vi "Start Rx.vi"(6 "error in (no error)":errorcluster, 8 "RX PARAMETER PANEL":T1={"Chain Mask"=0, "CF(MHz)"=2412, "CF2(MHz)"=0, "Data Rate"=0} {"Chain Mask" items=["0x1 : ch0"=1, "0x2 : ch1"=2, "0x4 : ch2"=4, "0x8 : ch3"=8, "0x3 : ch0, ch1"=3, "0x7 : ch0, ch1, ch2"=7, "0x15 : ch0, ch1, ch2, ch3"=15, "0x5 : ch0, ch2"=5, "0x10 : ch1, ch3"=10, "0x9 : ch1, ch3"=9, "0x12 : ch2, ch4"=12]; "Data Rate" items=["RATE_11B_LONG_1_MBPS"=0, "RATE_11B_LONG_2_MBPS"=1, "RATE_11B_LONG_5_5_MBPS"=2, "RATE_11B_LONG_11_MBPS"=3, "RATE_11B_SHORT_2_MBPS"=4, "RATE_11B_SHORT_5_5_MBPS"=5, "RATE_11B_SHORT_11_MBPS"=6, "RATE_11A_6_MBPS"=7, "RATE_11A_9_MBPS"=8, "RATE_11A_12_MBPS"=9, "RATE_11A_18_MBPS"=10, "RATE_11A_24_MBPS"=11, "RATE_11A_36_MBPS"=12, "RATE_11A_48_MBPS"=13, "RATE_11A_54_MBPS"=14, "RATE_11N_HT20_MCS0"=15, "RATE_11N_HT20_MCS1"=16, "RATE_11N_HT20_MCS2"=17, "RATE_11N_HT20_MCS3"=18, "RATE_11N_HT20_MCS4"=19, "RATE_11N_HT20_MCS5"=20, "RATE_11N_HT20_MCS6"=21, "RATE_11N_HT20_MCS7"=22, "RATE_11N_HT40_MCS0"=23, "RATE_11N_HT40_MCS1"=24, "RATE_11N_HT40_MCS2"=25, "RATE_11N_HT40_MCS3"=26, "RATE_11N_HT40_MCS4"=27, "RATE_11N_HT40_MCS5"=28, "RATE_11N_HT40_MCS6"=29, "RATE_11N_HT40_MCS7"=30, "RATE_11AC_HT20_MCS0"=31, "RATE_11AC_HT20_MCS1"=32, "RATE_11AC_HT20_MCS2"=33, "RATE_11AC_HT20_MCS3"=34, "RATE_11AC_HT20_MCS4"=35, "RATE_11AC_HT20_MCS5"=36, "RATE_11AC_HT20_MCS6"=37, "RATE_11AC_HT20_MCS7"=38, "RATE_11AC_HT20_MCS8"=39, "RATE_11AC_HT20_MCS9"=40, "RATE_11AC_HT40_MCS0"=41, "RATE_11AC_HT40_MCS1"=42, "RATE_11AC_HT40_MCS2"=43, "RATE_11AC_HT40_MCS3"=44, "RATE_11AC_HT40_MCS4"=45, "RATE_11AC_HT40_MCS5"=46, "RATE_11AC_HT40_MCS6"=47, "RATE_11AC_HT40_MCS7"=48, "RATE_11AC_HT40_MCS8"=49, "RATE_11AC_HT40_MCS9"=50, "RATE_11AC_HT80_MCS0"=51, "RATE_11AC_HT80_MCS1"=52, "RATE_11AC_HT80_MCS2"=53, "RATE_11AC_HT80_MCS3"=54, "RATE_11AC_HT80_MCS4"=55, "RATE_11AC_HT80_MCS5"=56, "RATE_11AC_HT80_MCS6"=57, "RATE_11AC_HT80_MCS7"=58, "RATE_11AC_HT80_MCS8"=59, "RATE_11AC_HT80_MCS9"=60, "RATE_11N_HT20_MCS8"=61, "RATE_11N_HT20_MCS9"=62, "RATE_11N_HT20_MCS10"=63, "RATE_11N_HT20_MCS11"=64, "RATE_11N_HT20_MCS12"=65, "RATE_11N_HT20_MCS13"=66, "RATE_11N_HT20_MCS14"=67, "RATE_11N_HT20_MCS15"=68, "RATE_11N_HT40_MCS8"=69, "RATE_11N_HT40_MCS9"=70, "RATE_11N_HT40_MCS10"=71, "RATE_11N_HT40_MCS11"=72, "RATE_11N_HT40_MCS12"=73, "RATE_11N_HT40_MCS13"=74, "RATE_11N_HT40_MCS14"=75, "RATE_11N_HT40_MCS15"=76, "RATE_11AC_HT20_MCS10"=77, "RATE_11AC_HT20_MCS11"=78, "RATE_11AC_HT20_MCS12"=79, "RATE_11AC_HT20_MCS13"=80, "RATE_11AC_HT20_MCS14"=81, "RATE_11AC_HT20_MCS15"=82, "RATE_11AC_HT20_MCS16"=83, "RATE_11AC_HT20_MCS17"=84, "RATE_11AC_HT20_MCS18"=85, "RATE_11AC_HT20_MCS19"=86, "RATE_11AC_HT40_MCS10"=87, "RATE_11AC_HT40_MCS11"=88, "RATE_11AC_HT40_MCS12"=89, "RATE_11AC_HT40_MCS13"=90, "RATE_11AC_HT40_MCS14"=91, "RATE_11AC_HT40_MCS15"=92, "RATE_11AC_HT40_MCS16"=93, "RATE_11AC_HT40_MCS17"=94, "RATE_11AC_HT40_MCS18"=95, "RATE_11AC_HT40_MCS19"=96, "RATE_11AC_HT80_MCS10"=97, "RATE_11AC_HT80_MCS11"=98, "RATE_11AC_HT80_MCS12"=99, "RATE_11AC_HT80_MCS13"=100, "RATE_11AC_HT80_MCS14"=101, "RATE_11AC_HT80_MCS15"=102, "RATE_11AC_HT80_MCS16"=103, "RATE_11AC_HT80_MCS17"=104, "RATE_11AC_HT80_MCS18"=105, "RATE_11AC_HT80_MCS19"=106, "RATE_11N_HT20_MCS16"=107, "RATE_11N_HT20_MCS17"=108, "RATE_11N_HT20_MCS18"=109, "RATE_11N_HT20_MCS19"=110, "RATE_11N_HT20_MCS20"=111, "RATE_11N_HT20_MCS21"=112, "RATE_11N_HT20_MCS22"=113, "RATE_11N_HT20_MCS23"=114, "RATE_11N_HT40_MCS16"=115, "RATE_11N_HT40_MCS17"=116, "RATE_11N_HT40_MCS18"=117, "RATE_11N_HT40_MCS19"=118, "RATE_11N_HT40_MCS20"=119, "RATE_11N_HT40_MCS21"=120, "RATE_11N_HT40_MCS22"=121, "RATE_11N_HT40_MCS23"=122, "RATE_11AC_HT20_MCS20"=123, "RATE_11AC_HT20_MCS21"=124, "RATE_11AC_HT20_MCS22"=125, "RATE_11AC_HT20_MCS23"=126, "RATE_11AC_HT20_MCS24"=127, "RATE_11AC_HT20_MCS25"=128, "RATE_11AC_HT20_MCS26"=129, "RATE_11AC_HT20_MCS27"=130, "RATE_11AC_HT20_MCS28"=131, "RATE_11AC_HT20_MCS29"=132, "RATE_11AC_HT40_MCS20"=133, "RATE_11AC_HT40_MCS21"=134, "RATE_11AC_HT40_MCS22"=135, "RATE_11AC_HT40_MCS23"=136, "RATE_11AC_HT40_MCS24"=137, "RATE_11AC_HT40_MCS25"=138, "RATE_11AC_HT40_MCS26"=139, "RATE_11AC_HT40_MCS27"=140, "RATE_11AC_HT40_MCS28"=141, "RATE_11AC_HT40_MCS29"=142, "RATE_11AC_HT80_MCS20"=143, "RATE_11AC_HT80_MCS21"=144, "RATE_11AC_HT80_MCS22"=145, "RATE_11AC_HT80_MCS23"=146, "RATE_11AC_HT80_MCS24"=147, "RATE_11AC_HT80_MCS25"=148, "RATE_11AC_HT80_MCS26"=149, "RATE_11AC_HT80_MCS27"=150, "RATE_11AC_HT80_MCS28"=151, "RATE_11AC_HT80_MCS29"=152, "RATE_11AC_HT20_MCS30"=153, "RATE_11AC_HT20_MCS31"=154, "RATE_11AC_HT20_MCS32"=155, "RATE_11AC_HT20_MCS33"=156, "RATE_11AC_HT20_MCS34"=157, "RATE_11AC_HT20_MCS35"=158, "RATE_11AC_HT20_MCS36"=159, "RATE_11AC_HT20_MCS37"=160, "RATE_11AC_HT20_MCS38"=161, "RATE_11AC_HT20_MCS39"=162, "RATE_11AC_HT40_MCS30"=163, "RATE_11AC_HT40_MCS31"=164, "RATE_11AC_HT40_MCS32"=165, "RATE_11AC_HT40_MCS33"=166, "RATE_11AC_HT40_MCS34"=167, "RATE_11AC_HT40_MCS35"=168, "RATE_11AC_HT40_MCS36"=169, "RATE_11AC_HT40_MCS37"=170, "RATE_11AC_HT40_MCS38"=171, "RATE_11AC_HT40_MCS39"=172, "RATE_11AC_HT80_MCS30"=173, "RATE_11AC_HT80_MCS31"=174, "RATE_11AC_HT80_MCS32"=175, "RATE_11AC_HT80_MCS33"=176, "RATE_11AC_HT80_MCS34"=177, "RATE_11AC_HT80_MCS35"=178, "RATE_11AC_HT80_MCS36"=179, "RATE_11AC_HT80_MCS37"=180, "RATE_11AC_HT80_MCS38"=181, "RATE_11AC_HT80_MCS39"=182, "RATE_11AC_HT160_MCS0"=183, "RATE_11AC_HT160_MCS1"=184, "RATE_11AC_HT160_MCS2"=185, "RATE_11AC_HT160_MCS3"=186, "RATE_11AC_HT160_MCS4"=187, "RATE_11AC_HT160_MCS5"=188, "RATE_11AC_HT160_MCS6"=189, "RATE_11AC_HT160_MCS7"=190, "RATE_11AC_HT160_MCS8"=191, "RATE_11AC_HT160_MCS9"=192, "RATE_11AC_HT160_MCS10"=193, "RATE_11AC_HT160_MCS11"=194, "RATE_11AC_HT160_MCS12"=195, "RATE_11AC_HT160_MCS13"=196, "RATE_11AC_HT160_MCS14"=197, "RATE_11AC_HT160_MCS15"=198, "RATE_11AC_HT160_MCS16"=199, "RATE_11AC_HT160_MCS17"=200, "RATE_11AC_HT160_MCS18"=201, "RATE_11AC_HT160_MCS19"=202, "RATE_11AC_HT160_MCS20"=203, "RATE_11AC_HT160_MCS21"=204, "RATE_11AC_HT160_MCS22"=205, "RATE_11AC_HT160_MCS23"=206, "RATE_11AC_HT160_MCS24"=207, "RATE_11AC_HT160_MCS25"=208, "RATE_11AC_HT160_MCS26"=209, "RATE_11AC_HT160_MCS27"=210, "RATE_11AC_HT160_MCS28"=211, "RATE_11AC_HT160_MCS29"=212, "RATE_11AC_HT160_MCS30"=213, "RATE_11AC_HT160_MCS31"=214, "RATE_11AC_HT160_MCS32"=215, "RATE_11AC_HT160_MCS33"=216, "RATE_11AC_HT160_MCS34"=217, "RATE_11AC_HT160_MCS35"=218, "RATE_11AC_HT160_MCS36"=219, "RATE_11AC_HT160_MCS37"=220, "RATE_11AC_HT160_MCS38"=221, "RATE_11AC_HT160_MCS39"=222, "RATE_11AC_HT80P80_MCS0"=223, "RATE_11AC_HT80P80_MCS1"=224, "RATE_11AC_HT80P80_MCS2"=225, "RATE_11AC_HT80P80_MCS3"=226, "RATE_11AC_HT80P80_MCS4"=227, "RATE_11AC_HT80P80_MCS5"=228, "RATE_11AC_HT80P80_MCS6"=229, "RATE_11AC_HT80P80_MCS7"=230, "RATE_11AC_HT80P80_MCS8"=231, "RATE_11AC_HT80P80_MCS9"=232, "RATE_11AC_HT80P80_MCS10"=233, "RATE_11AC_HT80P80_MCS11"=234, "RATE_11AC_HT80P80_MCS12"=235, "RATE_11AC_HT80P80_MCS13"=236, "RATE_11AC_HT80P80_MCS14"=237, "RATE_11AC_HT80P80_MCS15"=238, "RATE_11AC_HT80P80_MCS16"=239, "RATE_11AC_HT80P80_MCS17"=240, "RATE_11AC_HT80P80_MCS18"=241, "RATE_11AC_HT80P80_MCS19"=242, "RATE_11AC_HT80P80_MCS20"=243, "RATE_11AC_HT80P80_MCS21"=244, "RATE_11AC_HT80P80_MCS22"=245, "RATE_11AC_HT80P80_MCS23"=246, "RATE_11AC_HT80P80_MCS24"=247, "RATE_11AC_HT80P80_MCS25"=248, "RATE_11AC_HT80P80_MCS26"=249, "RATE_11AC_HT80P80_MCS27"=250, "RATE_11AC_HT80P80_MCS28"=251, "RATE_11AC_HT80P80_MCS29"=252, "RATE_11AC_HT80P80_MCS30"=253, "RATE_11AC_HT80P80_MCS31"=254, "RATE_11AC_HT80P80_MCS32"=255, "RATE_11AC_HT80P80_MCS33"=256, "RATE_11AC_HT80P80_MCS34"=257, "RATE_11AC_HT80P80_MCS35"=258, "RATE_11AC_HT80P80_MCS36"=259, "RATE_11AC_HT80P80_MCS37"=260, "RATE_11AC_HT80P80_MCS38"=261, "RATE_11AC_HT80P80_MCS39"=262, "RATE_11N_HT20_MCS24"=263, "RATE_11N_HT20_MCS25"=264, "RATE_11N_HT20_MCS26"=265, "RATE_11N_HT20_MCS27"=266, "RATE_11N_HT20_MCS28"=267, "RATE_11N_HT20_MCS29"=268, "RATE_11N_HT20_MCS30"=269, "RATE_11N_HT20_MCS31"=270, "RATE_11N_HT40_MCS24"=271, "RATE_11N_HT40_MCS25"=272, "RATE_11N_HT40_MCS26"=273, "RATE_11N_HT40_MCS27"=274, "RATE_11N_HT40_MCS28"=275, "RATE_11N_HT40_MCS29"=276, "RATE_11N_HT40_MCS30"=277, "RATE_11N_HT40_MCS31"=278, "RATE_11P_BW5_1p5_MBPS"=1007, "RATE_11P_BW5_2p25_MBPS"=1008, "RATE_11P_BW5_3_MBPS"=1009, "RATE_11P_BW5_4p5_MBPS"=1010, "RATE_11P_BW5_6_MBPS"=1011, "RATE_11P_BW5_9_MBPS"=1012, "RATE_11P_BW5_12_MBPS"=1013, "RATE_11P_BW5_13p5_MBPS"=1014, "RATE_11P_BW10_3_MBPS"=1107, "RATE_11P_BW10_4p5_MBPS"=1108, "RATE_11P_BW10_6_MBPS"=1109, "RATE_11P_BW10_9_MBPS"=1110, "RATE_11P_BW10_12_MBPS"=1111, "RATE_11P_BW10_18_MBPS"=1112, "RATE_11P_BW10_24_MBPS"=1113, "RATE_11P_BW10_27_MBPS"=1114, "RATE_11P_BW20_6_MBPS"=1207, "RATE_11P_BW20_9_MBPS"=1208, "RATE_11P_BW20_12_MBPS"=1209, "RATE_11P_BW20_18_MBPS"=1210, "RATE_11P_BW20_24_MBPS"=1211, "RATE_11P_BW20_36_MBPS"=1212, "RATE_11P_BW20_48_MBPS"=1213, "RATE_11P_BW20_54_MBPS"=1214]}, 9 "_hResourceContext":u32) -> (0 "error out":errorcluster, 2 "function return":bool, 3 "_hResourceContext out":u32)   [LabVIEW 2013, in "QCAWLAN_DLL.lvlib"]
doc: "QCA_DLL_Export bool StartRx(HANDLE _hResourceContext, int channel, int rxMode, int rateMask, int rxChain, int wlanMode, int channel2, int cbState);"
uses:
  QCAWLAN_DLL.lvlib
  TypeDef/RX PARAMETER PANEL.ctl
  TypeDef/CHAIN_MASK.ctl
  TypeDef/RX DATA RATE.ctl
  QCAWLAN_DLL.dll
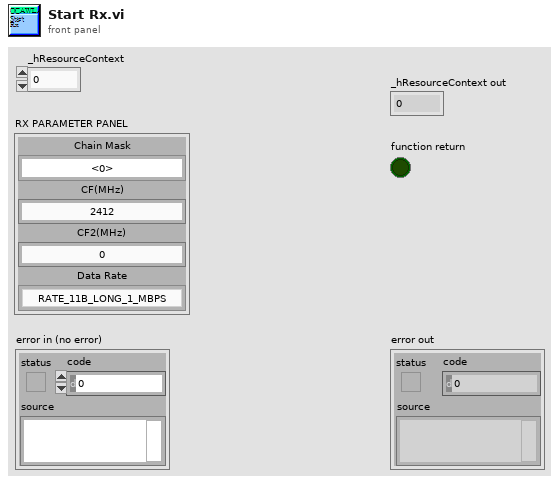
[diagram p1: front panel]
types:
  T1 = typedef "RX PARAMETER PANEL.ctl" = cluster{"Chain Mask":T2, "CF(MHz)":u32, "CF2(MHz)":u32, "Data Rate":T3}
  T2 = typedef "CHAIN_MASK.ctl" = u16
  T3 = typedef "RX DATA RATE.ctl" = u16
  T4 = typedef "CHANNEL BONDING STATE.ctl" = u16
  T5 = typedef "WLAN MODE.ctl" = u16
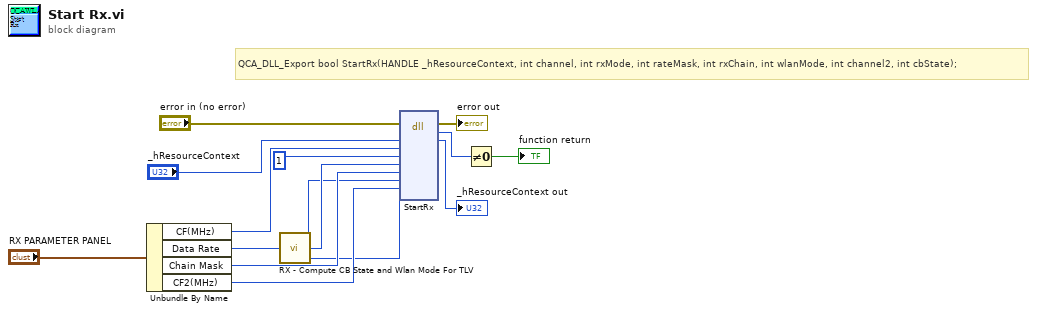
[diagram p0: block diagram]
diagram:
  # "QCA_DLL_Export bool StartRx(HANDLE _hResourceContext, int channel, int rxMode, int rateMask, int rxChain, int wlanMode, int channel2, int cbState);"
  n1 = Unbundle By Name("RX PARAMETER PANEL") -> ("CF(MHz)"=w8:u32, "Data Rate"=w7:T3, "Chain Mask"=w4:T2, "CF2(MHz)"=w2:u32)
  n2 = call "RX - Compute CB State and Wlan Mode For TLV.vi"("RX Data Rate"=w7) -> ("ChannelBondingState"=w1:T4, "RX Rate"=w5:i32, "WLAN Mode"=w3:T5)  [unwired: 2 in]
  n3 = dll-call lib="C:/Connectivity Client - MIMO/PlugIn/QCAWLAN_DLL.*" fn="StartRx"(error in="error in (no error)", "_hResourceContext"="_hResourceContext", "channel"=w8, "rxMode"=1, "rateMask"=w5, "rxChain"=w4, "wlanMode"=w3, "channel2"=w2, "cbState"=w1) -> (error out=→"error out":errorcluster, w14:u8, "_hResourceContext"=→"_hResourceContext out":u32)  [unwired: 9 in, 1 out]
  n4 = Not Equal To 0?(x=w14) -> (x != 0?=→"function return":bool)
